vi "PS_Sparker.vi"() -> (0 "error out":errorcluster)   [LabVIEW 2011]
uses:
  <vilib>/DAQmx/write.llb/DAQmx Write (Digital Bool 1Line 1Point).vi
  PS_Global.vi
  <vilib>/DAQmx/create/channels.llb/DAQmx Create Channel (DO-Digital Output).vi
  <vilib>/DAQmx/miscellaneous.llb/DAQmx Fill In Error Info.vi
panel:
  # "Run to spark"
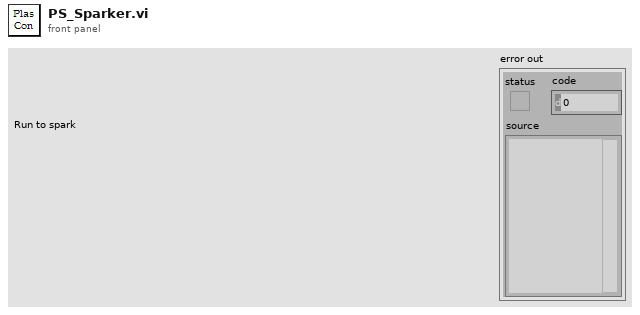
[diagram p1: front panel]
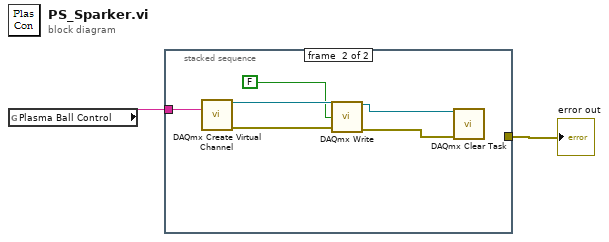
[diagram p0: block diagram]
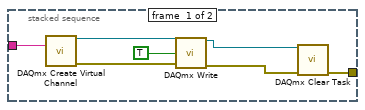
[diagram p2: hidden frame]
diagram:
  n1 = global read "PS_Global.vi" "Plasma Ball Control"() -> (w2:tag)
  n2 = stacked-sequence {
    tunnel: w2 -> [w9 w15]
    tunnel: [w4 _] -> w1
    frame #0 {
      n3 = call-poly <vilib>:"DAQmx Create Virtual Channel.vi"("lines"=w9) -> ("task out"=w8:refnum<k21>, "error out"=w7:errorcluster)  [unwired: 13 in]
      n4 = call-poly <vilib>:"DAQmx Write.vi"("task/channels in"=w8, "data"=TRUE, "error in"=w7) -> ("task out"=w6:refnum<k21>, "error out"=w5:errorcluster)  [unwired: 10 in, 1 out]
      n5 = call <vilib>:"DAQmx Clear Task.vi"("task in"=w6, "error in"=w5) -> ("error out"=w4:errorcluster)  [unwired: 13 in]
    }
    frame #1 {
      n6 = call-poly <vilib>:"DAQmx Create Virtual Channel.vi"("lines"=w15) -> ("task out"=w14:refnum<k21>, "error out"=w13:errorcluster)  [unwired: 13 in]
      n7 = call-poly <vilib>:"DAQmx Write.vi"("task/channels in"=w14, "data"=FALSE ("On/Off"), "error in"=w13) -> ("task out"=w12:refnum<k21>, "error out"=w11:errorcluster)  [unwired: 10 in, 1 out]
      n8 = call <vilib>:"DAQmx Clear Task.vi"("task in"=w12, "error in"=w11) -> ()  [unwired: 13 in, 1 out]
    }
  }
  "error out" <- w1
